vi "_ReadMethodFile.vi"(8 "error in (no error)":errorcluster, 11 "Path":path) -> (0 "error out":errorcluster, 3 "LVGetMethodXML":string)   [LabVIEW 2015]
uses:
  Y:/GitRepos on MAC/GitRepos/PerkinElmer/QRD-fw-server/Sniffer.900/External Dependencies/PerkinElmer.SimplicityServer.LVWrapper.dll
  External Dependencies/PerkinElmer.SimplicityServer.LVWrapper.dll
  <userlib>/_OpenG.lib/file/file.llb/Strip Path Extension - String__ogtk.vi
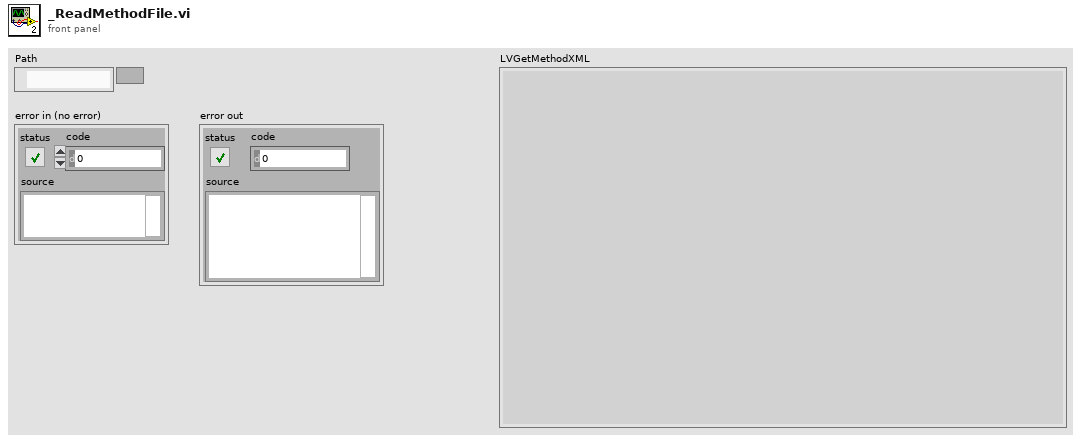
[diagram p1: front panel]
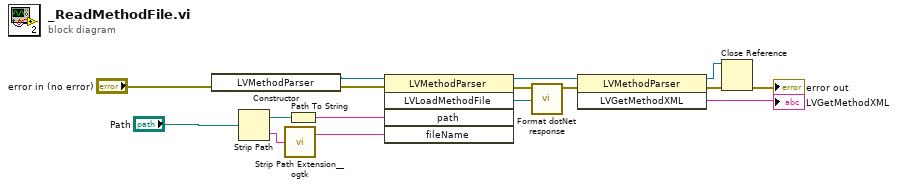
[diagram p0: block diagram]
diagram:
  n1 = constructor class="LVMethodParser"(error in="error in (no error)") -> (reference out=w2:refnum<k24>, error out=w3:errorcluster)  [unwired: 2 in, 1 out]
  n2 = Strip Path(path="Path") -> (stripped path=w8:path, name=w7:string)
  n3 = call-poly <userlib>:"Strip Path Extension__ogtk.vi"("path"=w7) -> ("root"=w12:string)  [unwired: 1 out]
  n4 = Path To String(path=w8) -> (string=w11:string)
  n5 = invoke class="LVMethodParser" method="LVLoadMethodFile"(reference=w2, error in=w3, "path"=w11, "fileName"=w12) -> (reference out=w13:refnum<k24>, error out=w5:errorcluster, "LVLoadMethodFile"=w6:refnum<k24>)  [unwired: 1 in, 2 out]
  n6 = call "Format dotNet response.vi"(".NET Refnum in"=w6, "error in (no error)"=w5) -> ("error IO"=w4:errorcluster)  [unwired: 9 in]
  n7 = invoke class="LVMethodParser" method="LVGetMethodXML"(reference=w13, error in=w4) -> (reference out=w14:refnum<k24>, error out=w15:errorcluster, "LVGetMethodXML"=→"LVGetMethodXML":string)  [unwired: 1 in]
  n8 = Close Reference(reference=w14, error in (no error)=w15) -> (error out=→"error out":errorcluster)
